vi "Process_abd_L.vi"(0 "Q_motor_in":refnum<queue>, 5 "출력 클러스터":T2, 7 "Control param In":T3={"L_velocity"=10000, "L_Power"=0.0, "R_velocity"=10000, "R_Power"=0.0, "T_param_L"={"Onset start"=0.0, "Onset end"=5.0, "Peak start"=10.0, "Release start"=60.0, "slang"=80.0, "Peak end"=58.0}, "T_param_R"={"Onset start"=0.0, "Onset end"=5.0, "Peak start"=10.0, "Release start"=60.0, "slang"=80.0, "Peak end"=58.0}, "Initialize?"=FALSE, "CAN read?"=FALSE, "Optimal count"=0}, 9 "Motor":T1, 11 "에러 입력(에러 없음)":errorcluster, 12 "Param In":T4) -> (4 "Q_motor_Out":refnum<queue>, 6 "Flag_L":T6(ring), 8 "GCP_1k_L":sgl, 10 "LOAD_CELL_PEAK_L":sgl[](array[numeric]), 13 "Control param out":T3, 14 "Param Out":T4, 15 "에러 출력":errorcluster)   [LabVIEW 2019]
uses:
  3b676039-217b-4c91-9efd-e0c48e4e0a54.vi
panel:
  in  "Process":T5={"LOAD_CELL_PEAK_L"=[12.0, 8.0], "LOAD_CELL_PEAK_R"=[], "Flag_L"=enum."Release_start", "Flag_R"=enum."Release_start", "Status_PS"="Init", "Q_data"={"Num_L"=0, "Period_L"=0, "GCP_L"=0.0, "Num_R"=0, "Period_R"=0, "GCP_R"=0.0, "FPGA_Data"=[], "L_RUN_OK"=FALSE, "R_RUN_OK"=FALSE, "L_ctrl_start"=FALSE, "R_ctrl_start"=FALSE, "Loop time"=0.0, "Integrated time"=0.0, "Mode"=enum."Negative"}}
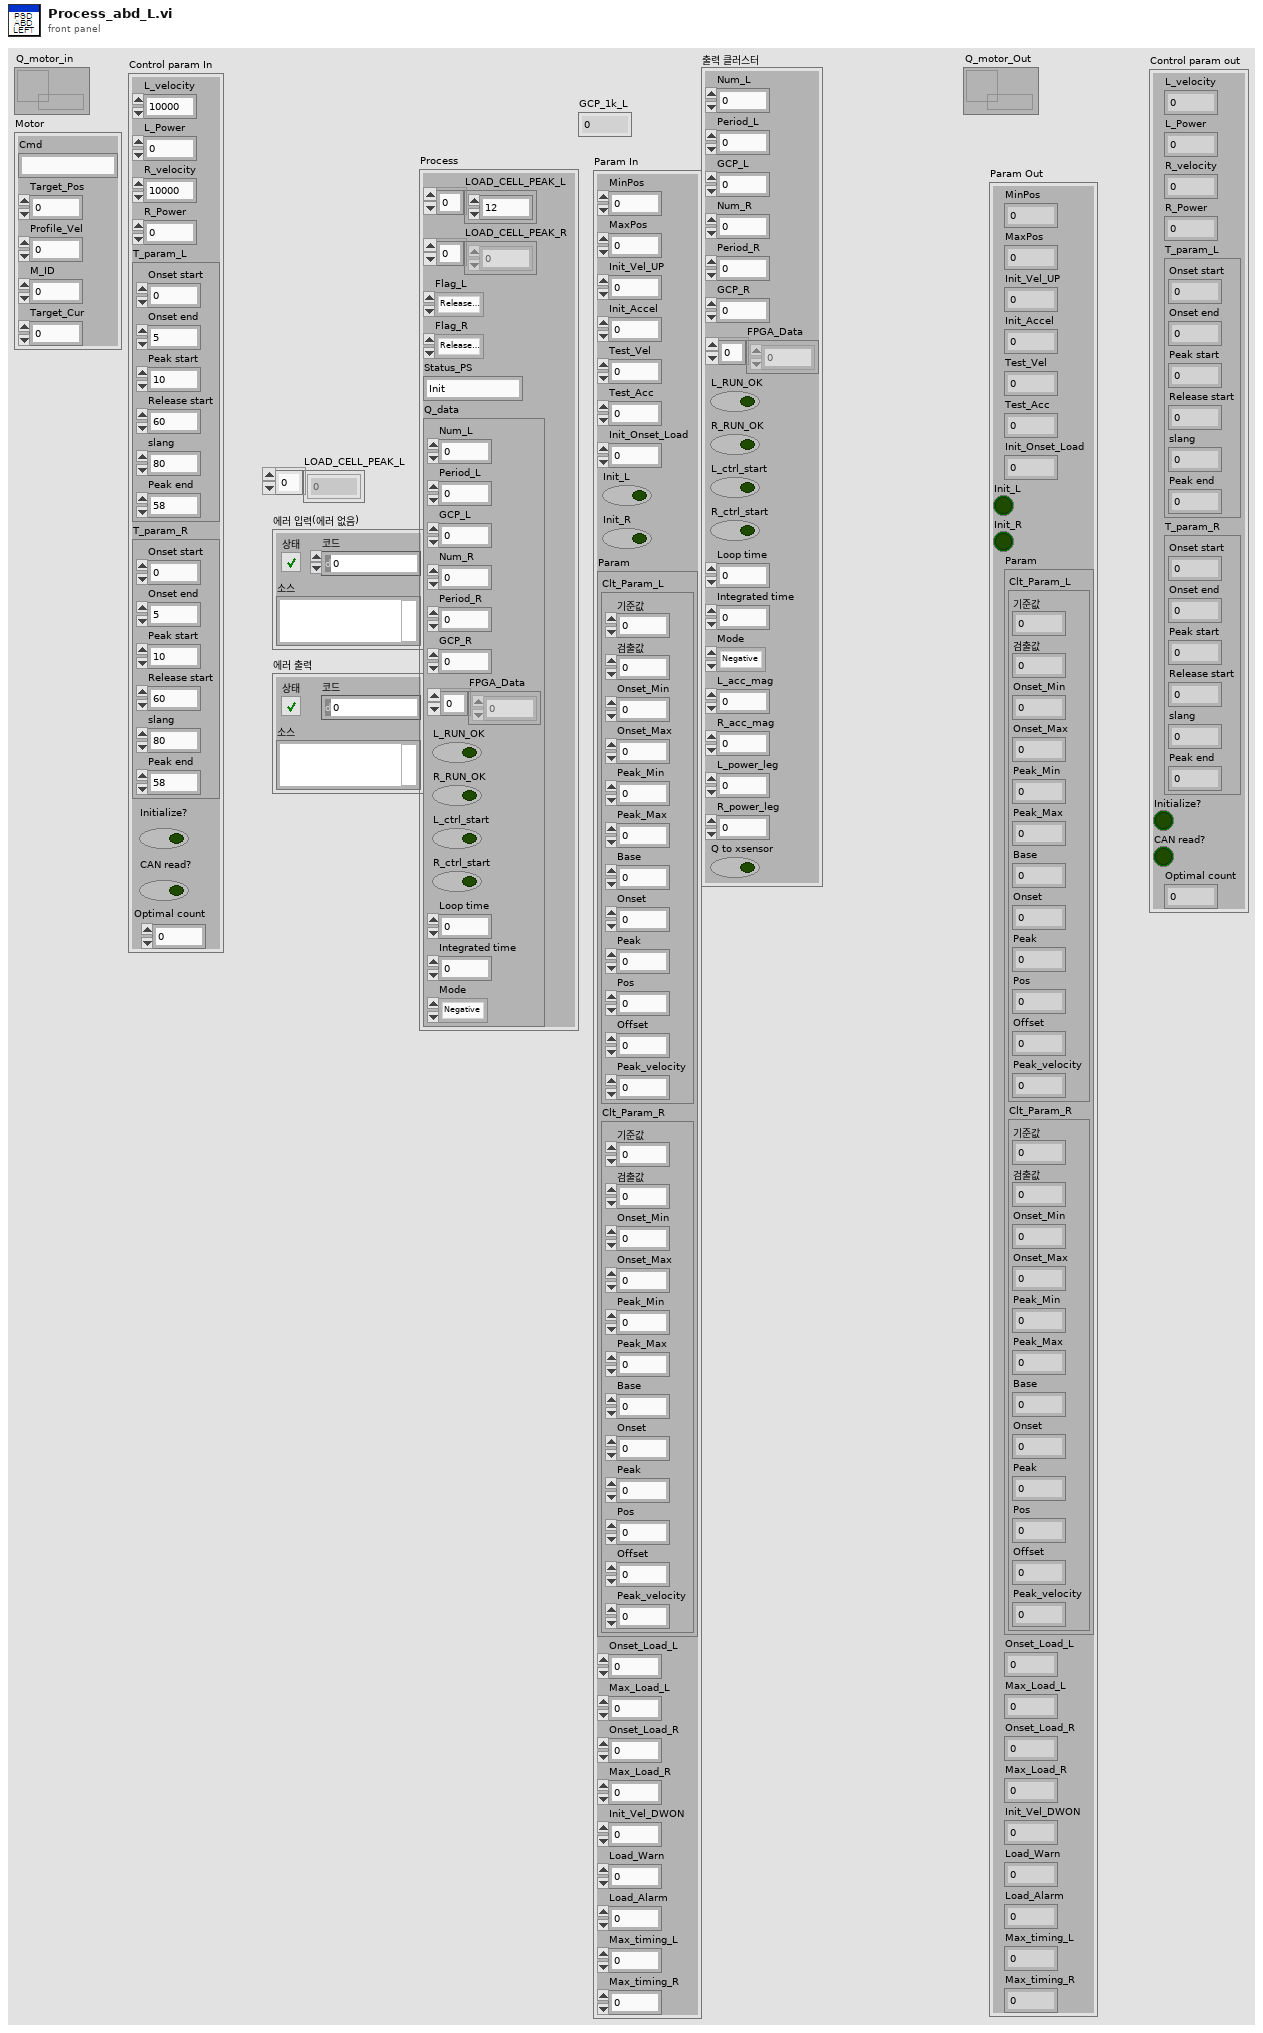
[diagram p1: front panel]
types:
  T1 = cluster{"Cmd":string, "Target_Pos":i32, "Profile_Vel":i32, "M_ID":u8, "Target_Cur":i32}
  T2 = cluster{"Num_L":u32, "Period_L":sgl, "GCP_L":sgl, "Num_R":u32, "Period_R":sgl, "GCP_R":sgl, "FPGA_Data":sgl[], "L_RUN_OK":bool, "R_RUN_OK":bool, "L_ctrl_start":bool, "R_ctrl_start":bool, "Loop time":dbl, "Integrated time":dbl, "Mode":enum16{"Negative", "Positive", "Full"}, "L_acc_mag":sgl, "R_acc_mag":sgl, "L_power_leg":sgl, "R_power_leg":sgl, "Q to xsensor":bool}
  T3 = cluster{"L_velocity":u32, "L_Power":sgl, "R_velocity":u32, "R_Power":sgl, "T_param_L":cluster{"Onset start":sgl, "Onset end":sgl, "Peak start":sgl, "Release start":sgl, "slang":sgl, "Peak end":sgl}, "T_param_R":cluster{"Onset start":sgl, "Onset end":sgl, "Peak start":sgl, "Release start":sgl, "slang":sgl, "Peak end":sgl}, "Initialize?":bool, "CAN read?":bool, "Optimal count":i32}
  T4 = cluster{"MinPos":i32, "MaxPos":i32, "Init_Vel_UP":i32, "Init_Accel":u32, "Test_Vel":i32, "Test_Acc":u32, "Init_Onset_Load":sgl, "Init_L":bool, "Init_R":bool, "Param":cluster{"Clt_Param_L":cluster{"기준값":sgl, "검출값":sgl, "Onset_Min":sgl, "Onset_Max":sgl, "Peak_Min":sgl, "Peak_Max":sgl, "Base":i32, "Onset":i32, "Peak":i32, "Pos":i32, "Offset":sgl, "Peak_velocity":i32}, "Clt_Param_R":cluster{"기준값":sgl, "검출값":sgl, "Onset_Min":sgl, "Onset_Max":sgl, "Peak_Min":sgl, "Peak_Max":sgl, "Base":i32, "Onset":i32, "Peak":i32, "Pos":i32, "Offset":sgl, "Peak_velocity":i32}}, "Onset_Load_L":sgl, "Max_Load_L":sgl, "Onset_Load_R":sgl, "Max_Load_R":sgl, "Init_Vel_DWON":i32, "Load_Warn":sgl, "Load_Alarm":sgl, "Max_timing_L":sgl, "Max_timing_R":sgl}
  T5 = cluster{"LOAD_CELL_PEAK_L":sgl[], "LOAD_CELL_PEAK_R":sgl[], "Flag_L":enum16{"Release_start", "Calculate", "Onset_start", "Peak_start"}, "Flag_R":enum16{"Release_start", "Calculate", "Onset_start", "Peak_start"}, "Status_PS":string, "Q_data":cluster{"Num_L":u32, "Period_L":u32, "GCP_L":sgl, "Num_R":u32, "Period_R":u32, "GCP_R":sgl, "FPGA_Data":sgl[], "L_RUN_OK":bool, "R_RUN_OK":bool, "L_ctrl_start":bool, "R_ctrl_start":bool, "Loop time":dbl, "Integrated time":dbl, "Mode":enum16{"Negative", "Positive", "Full"}}}
  T6 = enum16{"Release_start", "Calculate", "Onset_start", "Peak_start"}
  T7 = cluster{"Num_L":u32, "Period_L":sgl, "GCP_L":sgl, "Num_R":u32, "Period_R":sgl, "GCP_R":sgl, "FPGA_Data":sgl[], "L_RUN_OK":bool, "R_RUN_OK":bool, "L_ctrl_start":bool, "R_ctrl_start":bool, "Loop time":dbl, "Integrated time":dbl, "Mode":enum16{"Negative", "Positive", "Full"}, "L_acc_mag":sgl, "R_acc_mag":sgl, "L_power_leg":sgl, "R_power_leg":sgl}
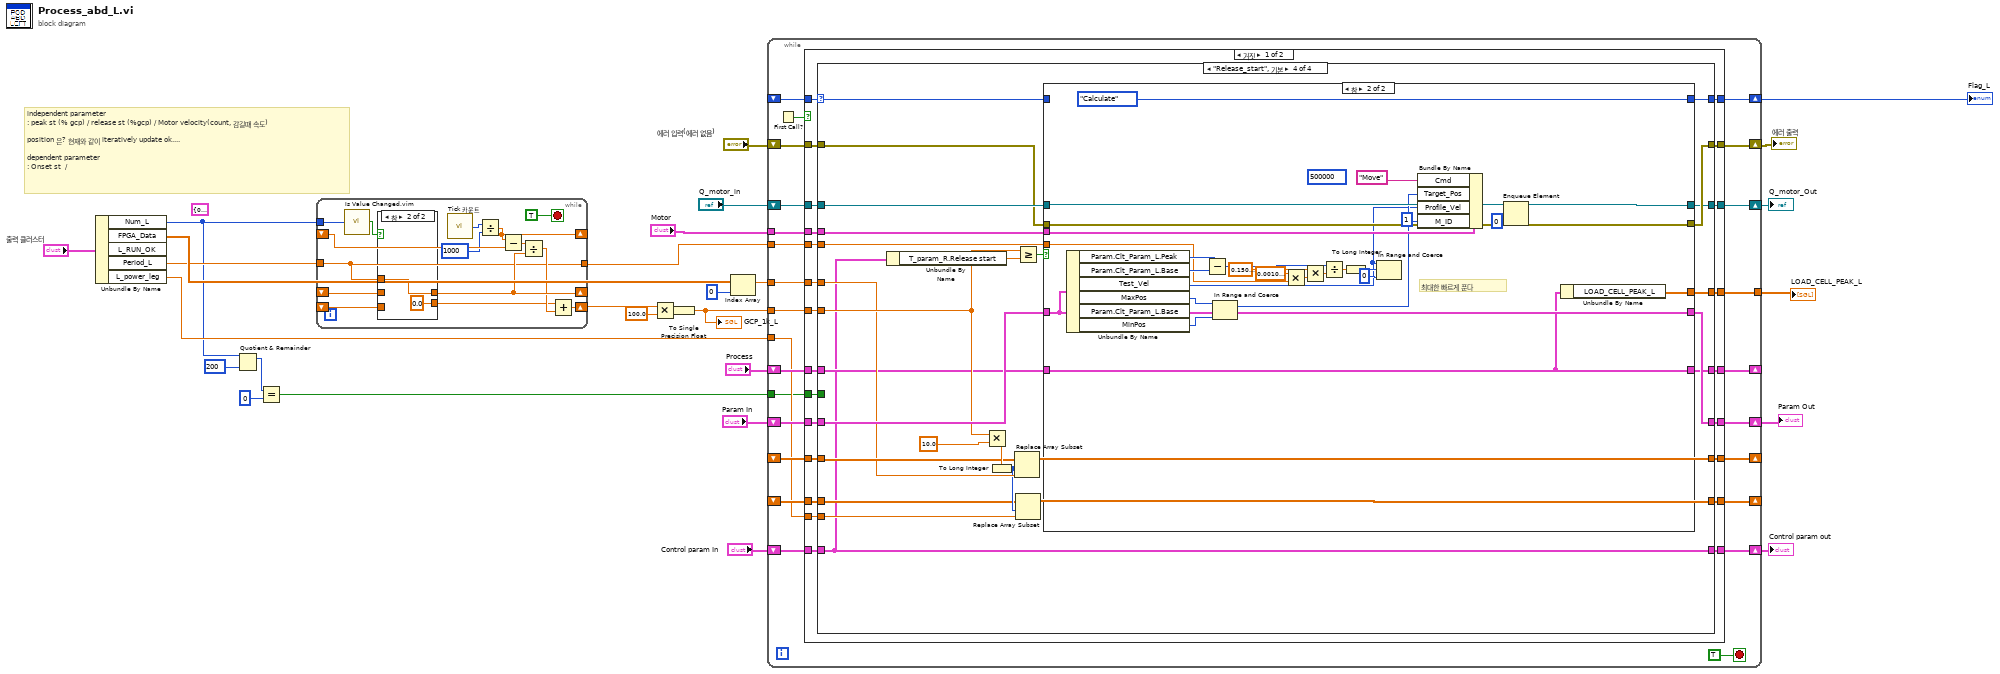
[diagram p0: block diagram]
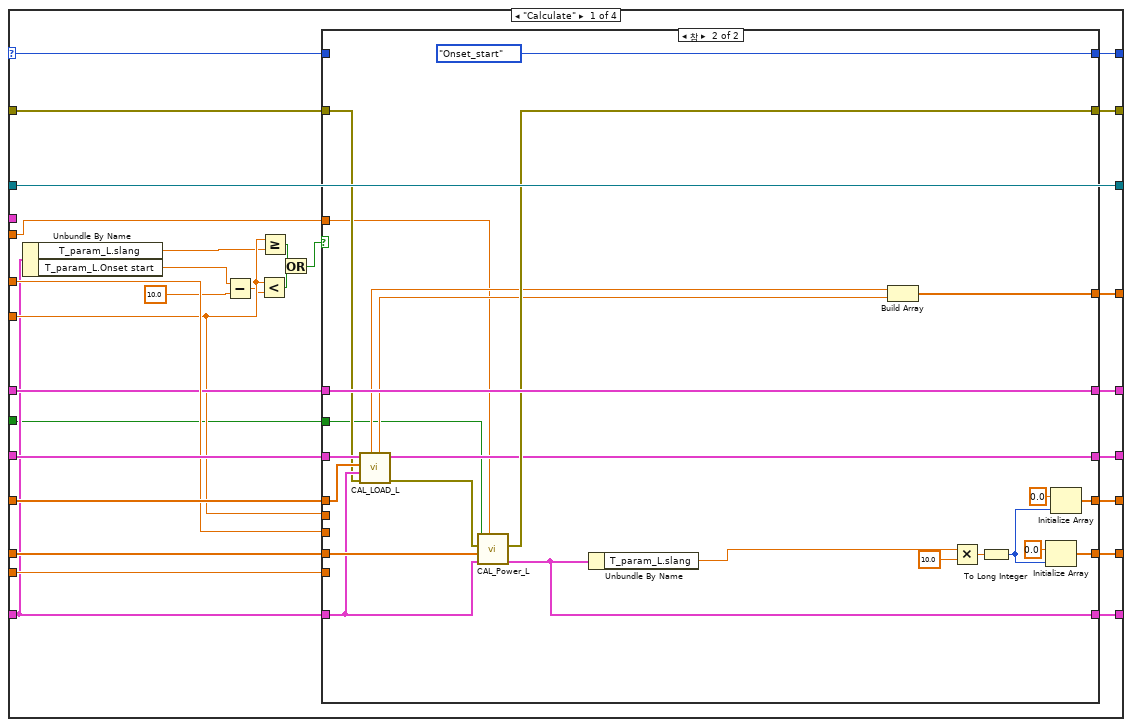
[diagram p3: hidden frame]
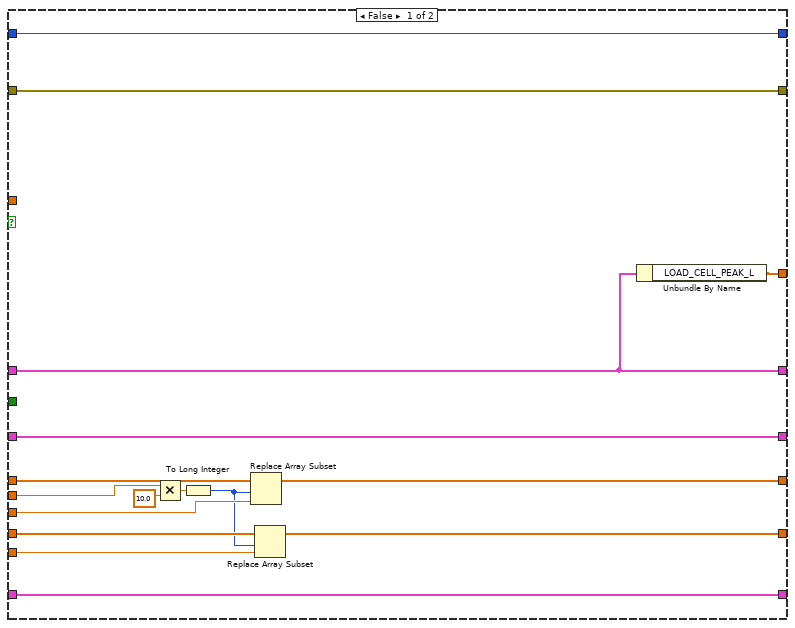
[diagram p4: hidden frame]
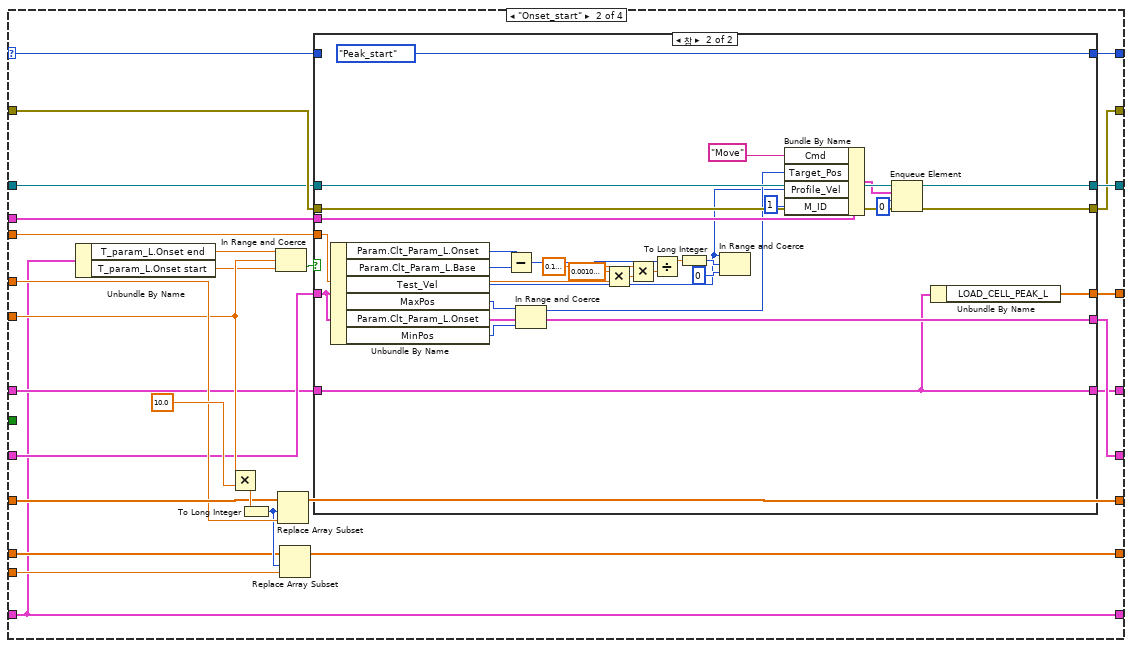
[diagram p5: hidden frame]
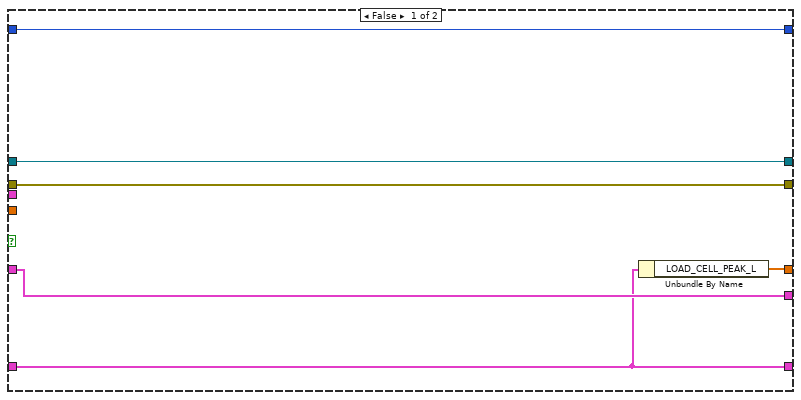
[diagram p6: hidden frame]
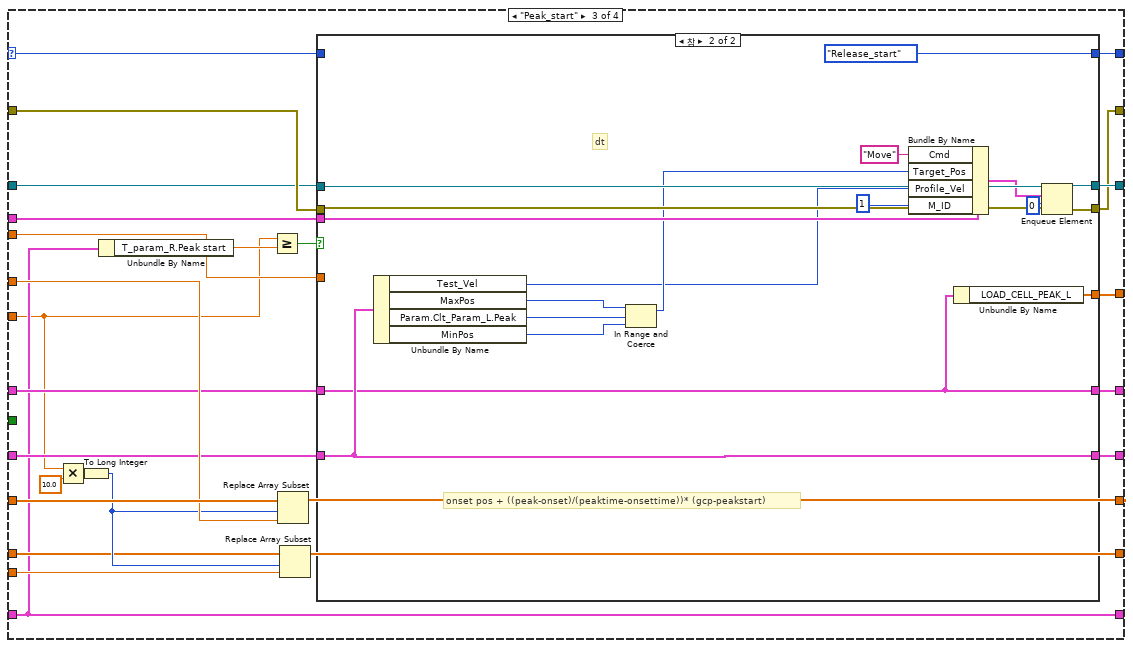
[diagram p7: hidden frame]
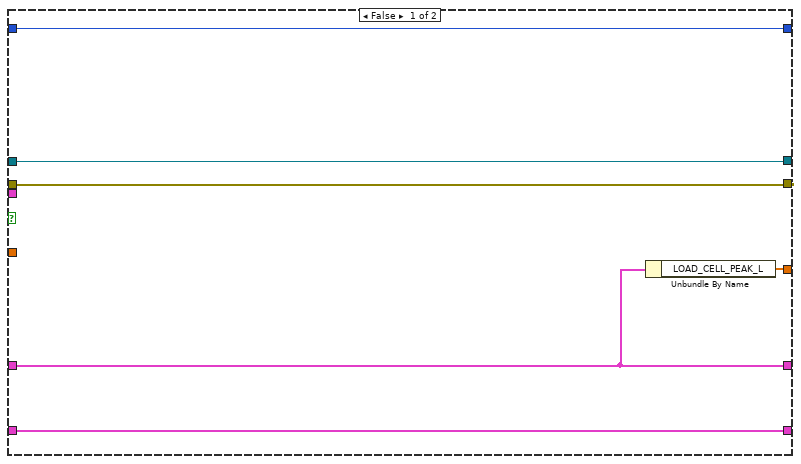
[diagram p8: hidden frame]
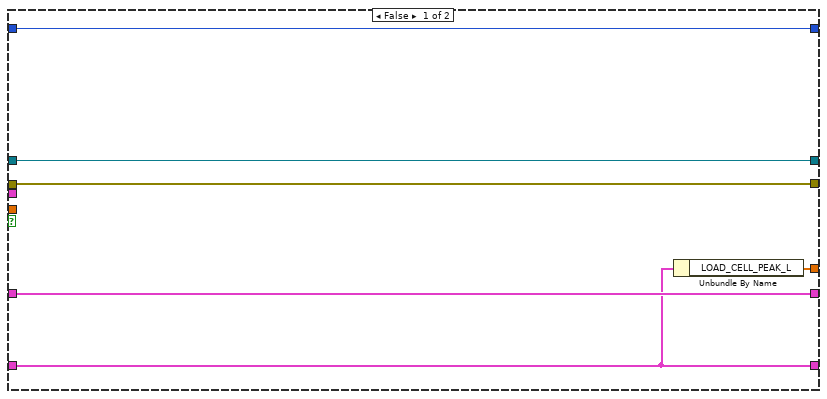
[diagram p9: hidden frame]
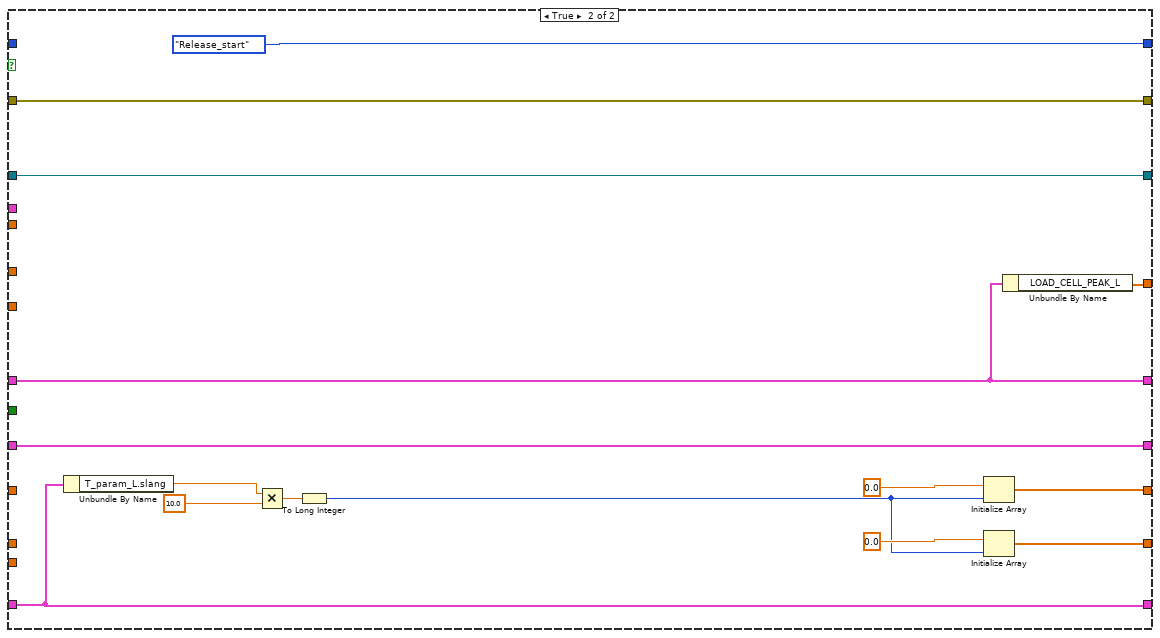
[diagram p10: hidden frame]
diagram:
  (unwired) T7 {"Num_L"=0, "Period_L"=0.0, "GCP_L"=0.0, "Num_R"=0, "Period_R"=0.0, "GCP_R"=0.0, "FPGA_Data"=[], "L_RUN_OK"=FALSE, "R_RUN_OK"=FALSE, "L_ctrl_start"=FALSE, "R_ctrl_start"=FALSE, "Loop time"=0.0, "Integrated time"=0.0, "Mode"=enum."Negative", "L_acc_mag"=0.0, "R_acc_mag"=0.0, "L_power_leg"=0.0, "R_power_leg"=0.0}
  # "independent parameter \n: peak st (% gcp) / release st (%gcp) / Motor velocity(count, 감길떄 속도) \n\nposition 은? 현재와 같이 iteratively update ok....  \n \ndependent parameter \n: Onset st  /"
  n1 = Unbundle By Name("출력 클러스터") -> ("Num_L"=w6:u32, "FPGA_Data"=w14:sgl[], "Period_L"=w13:sgl, "L_power_leg"=w15:sgl)  [unwired: 1 out]
  n2 = Quotient & Remainder(x=w6, y=u32 200) -> (x-y*floor(x/y)=w8:u32)  [unwired: 1 out]
  n3 = Equal?(x=w8, y=u32 0) -> (x = y?=w5:bool)
  n4 = while {
    shift-right: [w41] -> _
    shift-left: _ -> [w42]
    shift-right: [w39] -> w21
    shift-left: _ -> [w38]
    shift-right: [w32] -> _
    shift-left: _ -> [w35]
    tunnel: w13 -> [w29]
    tunnel: w6 -> [w31]
    tunnel: [w29] -> w12
    stop <- TRUE stop-if-true
    n5 = call "Is Value Changed.vim"("value"=w31) -> ("changed or first call?"=w30:bool)
    n6 = case shown="참" w30 {
      tunnel: w29 -> [_ w47]
      tunnel: [w45 w47] -> w41
      tunnel: w42 -> [w45 _]
      tunnel: w38 -> [w44 _]
      tunnel: [w44 0.0] -> w37
      frame False {
      }
      frame True {
      }
    }
    n7 = call "Tick 카운트"() -> ("Tick Count(uSec)"=w34:u32)
    n8 = Divide(x=w34, y=u32 1000) -> (x/y=w32:dbl)
    n9 = Subtract(x=w32, y=w35) -> (x-y=w36:dbl)
    n10 = Divide(x=w36, y=w41) -> (x/y=w40:dbl)
    n11 = Add(x=w37, y=w40) -> (x+y=w39:dbl)
  }
  n12 = Multiply(x=w21, y=100.0) -> (x*y=w19:dbl)
  n13 = To Single Precision Float(number=w19) -> (single precision float=w18:sgl)
  "GCP_1k_L" <- w18
  n14 = Index Array(array=w14, index=0 ("인덱스")) -> (element=w22:sgl)
  n15 = while {
    tunnel: [w70] -> w26
    tunnel: w12 -> [w66]
    tunnel: "Motor" -> [w63]
    tunnel: w22 -> [w61]
    tunnel: w18 -> [w60]
    shift-right: [w69] -> _
    shift-left: "Process" -> [w68]
    shift-right: [w72] -> w28
    shift-left: "에러 입력(에러 없음)" -> [w64]
    shift-right: [w67] -> w2
    shift-left: "Q_motor_in" -> [w62]
    shift-right: [w65] -> w16
    shift-left: "Param In" -> [w58]
    shift-right: [w71] -> w27
    shift-left: _ -> [w55]
    shift-right: [w57] -> _
    shift-left: _ -> [w59]
    shift-right: [w53] -> _
    shift-left: _ -> [w52]
    tunnel: w15 -> [w51]
    shift-right: [w50] -> w10
    shift-left: "Control param In" -> [w49]
    tunnel: w5 -> [w48]
    stop <- TRUE stop-if-true
    n16 = First Call?() -> (First Call?: T/F=w56:bool)
    n17 = case shown="거짓" w56 {
      tunnel: w55 -> [w95 _]
      tunnel: [w94 T6."Release_start"] -> w71
      tunnel: [w83 w348] -> w57
      tunnel: w58 -> [w93 w343]
      tunnel: w59 -> [w92 _]
      tunnel: w60 -> [w91 _]
      tunnel: w61 -> [w90 _]
      tunnel: w62 -> [w89 w347]
      tunnel: w63 -> [w88 _]
      tunnel: [w87 w347] -> w67
      tunnel: w64 -> [w86 w346]
      tunnel: [w85 w346] -> w72
      tunnel: [w84 w343] -> w65
      tunnel: w66 -> [w82 _]
      tunnel: [w81 w344] -> w70
      tunnel: w68 -> [w80 w345]
      tunnel: [w79 w345] -> w69
      tunnel: [w76 w338] -> w53
      tunnel: w52 -> [w78 _]
      tunnel: w51 -> [w77 _]
      tunnel: [w75 w337] -> w50
      tunnel: w49 -> [w74 w337]
      tunnel: w48 -> [w73 _]
      frame False {
        n18 = case shown="\"Release_start\", 기본" w95 {
          selector: w95 -> [w122 w189 w250 w300]
          tunnel: [w123 w190 w251 w301] -> w94
          tunnel: w93 -> [w120 w181 w238 w299]
          tunnel: w92 -> [w121 w186 w246 w294]
          tunnel: w91 -> [w109 w183 w226 w296]
          tunnel: w90 -> [w118 w185 w245 w293]
          tunnel: w89 -> [w117 w174 w236 w292]
          tunnel: w88 -> [_ w179 w242 w291]
          tunnel: [w117 w177 w241 w285] -> w87
          tunnel: w86 -> [w116 w178 w243 w290]
          tunnel: [w113 w176 w240 w289] -> w85
          tunnel: [w119 w180 w237 w287] -> w84
          tunnel: [w115 w182 w244 w288] -> w83
          tunnel: w82 -> [w97 w175 w239 w286]
          tunnel: [w114 w173 w235 w284] -> w81
          tunnel: w80 -> [w112 w172 w234 w283]
          tunnel: [w111 w171 w233 w282] -> w79
          tunnel: w78 -> [w104 w169 w231 w280]
          tunnel: w77 -> [w103 w168 w230 w279]
          tunnel: [w102 w167 w229 w278] -> w76
          tunnel: [w101 w164 w227 w276] -> w75
          tunnel: w74 -> [w100 w164 w227 w276]
          tunnel: w73 -> [w96 _ _ _]
          frame "Calculate" {
            n19 = Unbundle By Name(w100) -> ("T_param_L.slang"=w98:sgl, "T_param_L.Onset start"=w99:sgl)
            n20 = Subtract(x=w99, y=sgl 10.0) -> (x-y=w108:sgl)
            n21 = Less?(x=w109, y=w108) -> (x < y?=w106:bool)
            n22 = Greater Or Equal?(x=w109, y=w98) -> (x >= y?=w107:bool)
            n23 = Or(x=w107, y=w106) -> (x .or. y?=w105:bool)
            n24 = case shown="참" w105 {
              tunnel: [w139 T6."Onset_start"] -> w123
              tunnel: w122 -> [w139 _]
              tunnel: w121 -> [w138 w147]
              tunnel: w120 -> [w133 w149]
              tunnel: [w133 w148] -> w119
              tunnel: w118 -> [w137 _]
              tunnel: w109 -> [w134 _]
              tunnel: [w129 w161] -> w115
              tunnel: w116 -> [w132 w143]
              tunnel: [w132 w150] -> w113
              tunnel: [w130 w160] -> w114
              tunnel: w112 -> [w131 w159]
              tunnel: [w131 w159] -> w111
              tunnel: w104 -> [w128 w153]
              tunnel: w103 -> [w126 _]
              tunnel: [w125 w157] -> w102
              tunnel: [w124 w151] -> w101
              tunnel: w100 -> [w124 w146]
              tunnel: w97 -> [_ w141]
              tunnel: w96 -> [_ w140]
              frame False {
                n25 = Multiply(x=w134, y=10.0) -> (x*y=w136:dbl)
                n26 = To Long Integer(number=w136) -> (32bit integer=w127:i32)
                n27 = Replace Array Subset(array=w138, new element=w137, index=w127) -> (w129:sgl[])
                n28 = Replace Array Subset(array=w128, new element=w126, index=w127) -> (w125:sgl[])
                n29 = Unbundle By Name(w131) -> ("LOAD_CELL_PEAK_L"=w130:sgl[])
              }
              frame True {
                n30 = call "CAL_LOAD_L.vi"("Param In"=w149, "Force"=w147, "Control param In"=w146, "에러 입력(에러 없음) 2"=w143) -> ("Load_Onset"=w144:sgl, "Load_Peak"=w145:sgl, "Param Out"=w148:T4, "에러 입력(에러 없음) 3"=w142:errorcluster)  [unwired: 3 in]
                n31 = call "CAL_Power_L.vi"("stride?"=w140, "에러 입력(에러 없음)"=w142, "Positive Power"=w153, "Control param In"=w146, "Period_L"=w141) -> ("에러 출력"=w150:errorcluster, "Control param out"=w151:T3)  [unwired: 4 in]
                n32 = Unbundle By Name(w151) -> ("T_param_L.slang"=w152:sgl)
                n33 = Build Array(w144, w145) -> (w160:sgl[])
                n34 = Multiply(x=w152, y=sgl 10.0) -> (x*y=w155:sgl)
                n35 = To Long Integer(number=w155) -> (32bit integer=w154:i32)
                n36 = Initialize Array(sgl 0.0 ("원소"), w154) -> (w157:sgl[])
                n37 = Initialize Array(sgl 0.0 ("원소"), w154) -> (w161:sgl[])
              }
            }
          }
          frame "Onset_start" {
            n38 = Unbundle By Name(w164) -> ("T_param_L.Onset end"=w166:sgl, "T_param_L.Onset start"=w165:sgl)
            n39 = Multiply(x=w183, y=10.0) -> (x*y=w187:dbl)
            n40 = To Long Integer(number=w187) -> (32bit integer=w170:i32)
            n41 = In Range and Coerce(upper limit=w166, x=w183, lower limit=w165) -> (In Range?=w184:bool)  [unwired: 1 out]
            n42 = Replace Array Subset(array=w186, new element=w185, index=w170) -> (w182:sgl[])
            n43 = Replace Array Subset(array=w169, new element=w168, index=w170) -> (w167:sgl[])
            n44 = case shown="참" w184 {
              tunnel: [w196 T6."Peak_start"] -> w190
              tunnel: w189 -> [w196 _]
              tunnel: w181 -> [w194 w211]
              tunnel: [w194 w211] -> w180
              tunnel: w179 -> [_ w210]
              tunnel: w178 -> [w193 w201]
              tunnel: w174 -> [w195 w209]
              tunnel: [w195 w200] -> w177
              tunnel: [w193 w199] -> w176
              tunnel: w175 -> [_ w208]
              tunnel: [w191 w202] -> w173
              tunnel: [w192 w203] -> w171
              tunnel: w172 -> [w192 w203]
              frame False {
                n45 = Unbundle By Name(w192) -> ("LOAD_CELL_PEAK_L"=w191:sgl[])
              }
              frame True {
                n46 = Unbundle By Name(w211) -> ("Param.Clt_Param_L.Onset"=w218:i32, "Param.Clt_Param_L.Base"=w217:i32, "Test_Vel"=w197:i32, "MaxPos"=w216:i32, "Param.Clt_Param_L.Onset"=w204:i32, "MinPos"=w215:i32)
                n47 = Subtract(x=w218, y=w217) -> (x-y=w224:i32)
                n48 = In Range and Coerce(upper limit=w216, x=w204, lower limit=w215) -> (coerced(x)=w198:i32)  [unwired: 1 out]
                n49 = Multiply(x=sgl 0.001 ("y"), y=w208) -> (x*y=w222:sgl)
                n50 = Multiply(x=sgl 0.1 ("y"), y=w222) -> (x*y=w225:sgl)
                n51 = Divide(x=w224, y=w225) -> (x/y=w205:sgl)
                n52 = To Long Integer(number=w205) -> (32bit integer=w223:i32)
                n53 = In Range and Coerce(upper limit=w197, x=w223, lower limit=0) -> ()  [unwired: 2 out]
                n54 = Bundle By Name(cluster=w210, "Cmd"="Move", "Target_Pos"=w198, "Profile_Vel"=w197, "M_ID"=u8 1) -> (w207:T1)
                n55 = Enqueue Element(queue=w209, element=w207, timeout in ms (-1)=0 ("타임아웃(ms) (-1)"), error in (no error)=w201) -> (queue out=w200:refnum<queue>, error out=w199:errorcluster)  [unwired: 1 out]
                n56 = Unbundle By Name(w203) -> ("LOAD_CELL_PEAK_L"=w202:sgl[])
              }
            }
          }
          frame "Peak_start" {
            n57 = Multiply(x=w226, y=10.0) -> (x*y=w248:dbl)
            n58 = To Long Integer(number=w248) -> (32bit integer=w232:i32)
            n59 = Unbundle By Name(w227) -> ("T_param_R.Peak start"=w228:sgl)
            n60 = Greater Or Equal?(x=w226, y=w228) -> (x >= y?=w247:bool)
            n61 = Replace Array Subset(array=w246, new element=w245, index=w232) -> (w244:sgl[])
            n62 = Replace Array Subset(array=w231, new element=w230, index=w232) -> (w229:sgl[])
            n63 = case shown="참" w247 {
              tunnel: [w257 T6."Release_start"] -> w251
              tunnel: w250 -> [w257 _]
              tunnel: w236 -> [w256 w270]
              tunnel: w243 -> [w254 w265]
              tunnel: w242 -> [_ w269]
              tunnel: [w256 w261] -> w241
              tunnel: [w254 w262] -> w240
              tunnel: w239 -> [_ _]
              tunnel: w238 -> [w255 w268]
              tunnel: [w255 w268] -> w237
              tunnel: [w252 w263] -> w235
              tunnel: w234 -> [w253 w264]
              tunnel: [w253 w264] -> w233
              frame False {
                n64 = Unbundle By Name(w253) -> ("LOAD_CELL_PEAK_L"=w252:sgl[])
              }
              frame True {
                # "onset pos + ((peak-onset)/(peaktime-onsettime))* (gcp-peakstart)"
                # "dt"
                n65 = Unbundle By Name(w268) -> ("Test_Vel"=w258:i32, "MaxPos"=w275:i32, "Param.Clt_Param_L.Peak"=w266:i32, "MinPos"=w274:i32)
                n66 = In Range and Coerce(upper limit=w275, x=w266, lower limit=w274) -> (coerced(x)=w260:i32)  [unwired: 1 out]
                n67 = Bundle By Name(cluster=w269, "Cmd"="Move", "Target_Pos"=w260, "Profile_Vel"=w258, "M_ID"=u8 1) -> (w267:T1)
                n68 = Unbundle By Name(w264) -> ("LOAD_CELL_PEAK_L"=w263:sgl[])
                n69 = Enqueue Element(queue=w270, element=w267, timeout in ms (-1)=0 ("타임아웃(ms) (-1)"), error in (no error)=w265) -> (queue out=w261:refnum<queue>, error out=w262:errorcluster)  [unwired: 1 out]
              }
            }
          }
          frame "Release_start", Default {
            n70 = Unbundle By Name(w276) -> ("T_param_R.Release start"=w277:sgl)
            n71 = Multiply(x=w296, y=10.0) -> (x*y=w295:dbl)
            n72 = To Long Integer(number=w295) -> (32bit integer=w281:i32)
            n73 = Replace Array Subset(array=w294, new element=w293, index=w281) -> (w288:sgl[])
            n74 = Greater Or Equal?(x=w296, y=w277) -> (x >= y?=w298:bool)
            n75 = Replace Array Subset(array=w280, new element=w279, index=w281) -> (w278:sgl[])
            n76 = case shown="참" w298 {
              tunnel: [w307 T6."Calculate"] -> w301
              tunnel: w300 -> [w307 _]
              tunnel: w299 -> [w305 w320]
              tunnel: w292 -> [w306 w318]
              tunnel: w291 -> [_ w321]
              tunnel: [w306 w310] -> w285
              tunnel: w290 -> [w304 w311]
              tunnel: [w304 w309] -> w289
              tunnel: [w305 w320] -> w287
              tunnel: w286 -> [_ w319]
              tunnel: [w303 w313] -> w284
              tunnel: w283 -> [w302 w312]
              tunnel: [w302 w312] -> w282
              frame False {
                n77 = Unbundle By Name(w302) -> ("LOAD_CELL_PEAK_L"=w303:sgl[])
              }
              frame True {
                (unwired) 500000 ("Profile_Vel")
                # "최대한 빠르게 푼다"
                n78 = Unbundle By Name(w320) -> ("Param.Clt_Param_L.Peak"=w328:i32, "Param.Clt_Param_L.Base"=w327:i32, "Test_Vel"=w308:i32, "MaxPos"=w326:i32, "Param.Clt_Param_L.Base"=w315:i32, "MinPos"=w325:i32)
                n79 = Subtract(x=w328, y=w327) -> (x-y=w334:i32)
                n80 = In Range and Coerce(upper limit=w326, x=w315, lower limit=w325) -> (coerced(x)=w314:i32)  [unwired: 1 out]
                n81 = Multiply(x=sgl 0.001 ("y"), y=w319) -> (x*y=w332:sgl)
                n82 = Multiply(x=sgl 0.15 ("y"), y=w332) -> (x*y=w335:sgl)
                n83 = Divide(x=w334, y=w335) -> (x/y=w316:sgl)
                n84 = To Long Integer(number=w316) -> (32bit integer=w333:i32)
                n85 = In Range and Coerce(upper limit=w308, x=w333, lower limit=0) -> ()  [unwired: 2 out]
                n86 = Bundle By Name(cluster=w321, "Cmd"="Move", "Target_Pos"=w314, "Profile_Vel"=w308, "M_ID"=u8 1) -> ()  [unwired: 1 out]
                n87 = Enqueue Element(queue=w318, timeout in ms (-1)=0 ("타임아웃(ms) (-1)"), error in (no error)=w311) -> (queue out=w310:refnum<queue>, error out=w309:errorcluster)  [unwired: 1 in, 1 out]
                n88 = Unbundle By Name(w312) -> ("LOAD_CELL_PEAK_L"=w313:sgl[])
              }
            }
          }
        }
      }
      frame True {
        n89 = Unbundle By Name(w337) -> ("T_param_L.slang"=w336:sgl)
        n90 = Multiply(x=w336, y=sgl 10.0) -> (x*y=w341:sgl)
        n91 = To Long Integer(number=w341) -> (32bit integer=w339:i32)
        n92 = Initialize Array(sgl 0.0 ("원소"), w339) -> (w348:sgl[])
        n93 = Initialize Array(sgl 0.0 ("원소"), w339) -> (w338:sgl[])
        n94 = Unbundle By Name(w345) -> ("LOAD_CELL_PEAK_L"=w344:sgl[])
      }
    }
  }
  "에러 출력" <- w28
  "Flag_L" <- w27
  "LOAD_CELL_PEAK_L" <- w26
  "Param Out" <- w16
  "Control param out" <- w10
  "Q_motor_Out" <- w2
